vi "Code Migration Paths.vi"(11 "error in (no error)":errorcluster) -> (2 "Folders to Ignore":path, 3 "Deafult value setter VI":path, 4 "IS Project Directory":path, 6 "IO Controls":path, 8 "Get Resource VI":path, 10 "Error Log Path":path, 13 "Deserializer":path, 14 "Serializer":path, 15 "error out":errorcluster)   [LabVIEW 2021, in "Path Functions.lvlib"]
uses:
  Path Functions.lvlib
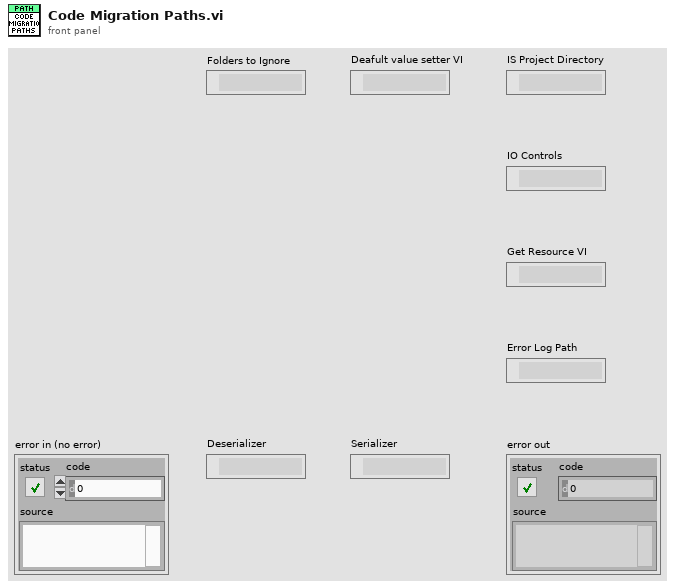
[diagram p1: front panel]
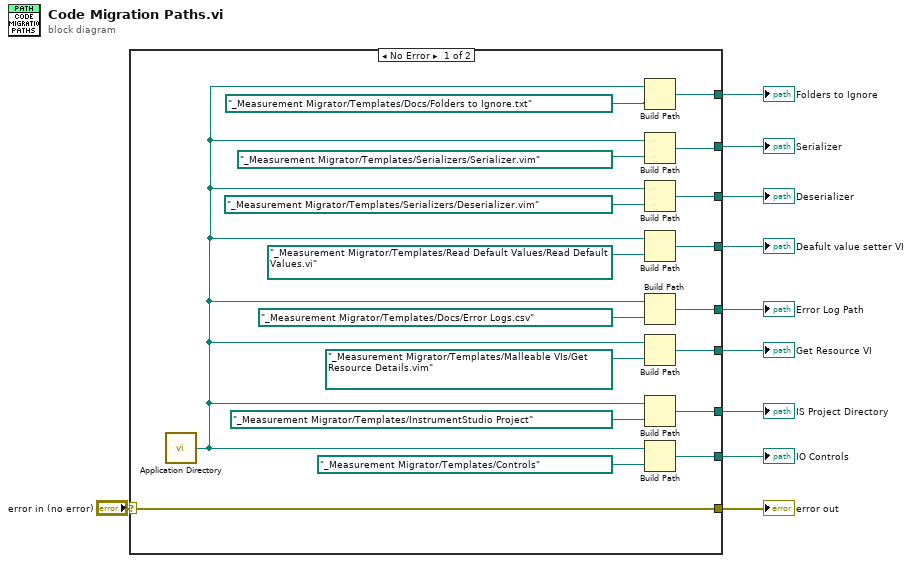
[diagram p0: block diagram]
diagram:
  n1 = case shown="No Error" "error in (no error)" {
    selector: "error in (no error)" -> [w20 w29]
    tunnel: [w27 _] -> w10
    tunnel: [w25 _] -> w9
    tunnel: [w24 _] -> w8
    tunnel: [w21 _] -> w7
    tunnel: [w14 _] -> w6
    tunnel: [w20 w29] -> w5
    tunnel: [w17 _] -> w3
    tunnel: [w15 _] -> w2
    tunnel: [w11 _] -> w1
    frame No Error {
      n2 = call <vilib>:"Application Directory.vi"() -> ("Application Directory"=w13:path)
      n3 = Build Path(base path=w13, name or relative path=path "_Measurement Migrator/Templates/Docs/Folders to Ignore.txt") -> (appended path=w11:path)
      n4 = Build Path(base path=w13, name or relative path=path "_Measurement Migrator/Templates/Serializers/Serializer.vim") -> (appended path=w14:path)
      n5 = Build Path(base path=w13, name or relative path=path "_Measurement Migrator/Templates/Serializers/Deserializer.vim") -> (appended path=w17:path)
      n6 = Build Path(base path=w13, name or relative path=path "_Measurement Migrator/Templates/Read Default Values/Read Default Values.vi") -> (appended path=w15:path)
      n7 = Build Path(base path=w13, name or relative path=path "_Measurement Migrator/Templates/Docs/Error Logs.csv") -> (appended path=w21:path)
      n8 = Build Path(base path=w13, name or relative path=path "_Measurement Migrator/Templates/Malleable VIs/Get Resource Details.vim") -> (appended path=w24:path)
      n9 = Build Path(base path=w13, name or relative path=path "_Measurement Migrator/Templates/InstrumentStudio Project") -> (appended path=w27:path)
      n10 = Build Path(base path=w13, name or relative path=path "_Measurement Migrator/Templates/Controls") -> (appended path=w25:path)
    }
    frame Error {
    }
  }
  "error out" <- w5
  "IS Project Directory" <- w10
  "IO Controls" <- w9
  "Get Resource VI" <- w8
  "Error Log Path" <- w7
  "Deserializer" <- w3
  "Serializer" <- w6
  "Deafult value setter VI" <- w2
  "Folders to Ignore" <- w1
